vi "VFH Visualization.vi"() -> ()   [LabVIEW 2011]
uses:
  <vilib>/Platform/TimedLoop/XDataNode/timing_clust.ctl
  <vilib>/Platform/TimedLoop/XDataNode/nitl_modes.ctl
  <vilib>/Platform/TimedLoop/XDataNode/wakeup.ctl
  <vilib>/Platform/TimedLoop/XDataNode/XDataNode.xnode
  <vilib>/Platform/TimedLoop/XDataNode/XDNodeRunTimeDep.lvlib
  <vilib>/Analysis/NI_AALPro.lvlib
  <vilib>/Analysis/coordinate.llb/2D Cartesian Coordinate Rotation (Array).vi
  <vilib>/Analysis/NI_AAL_Angle.lvlib
  <vilib>/Analysis/coordinate.llb/Wrap Angle (scalar).vi
panel:
  in  "stop?":bool
  out "VY History":dbl(graph)
  out "Heading History":dbl(graph)
  out "LIDAR data":cluster{dbl[], dbl[]}[](graph)
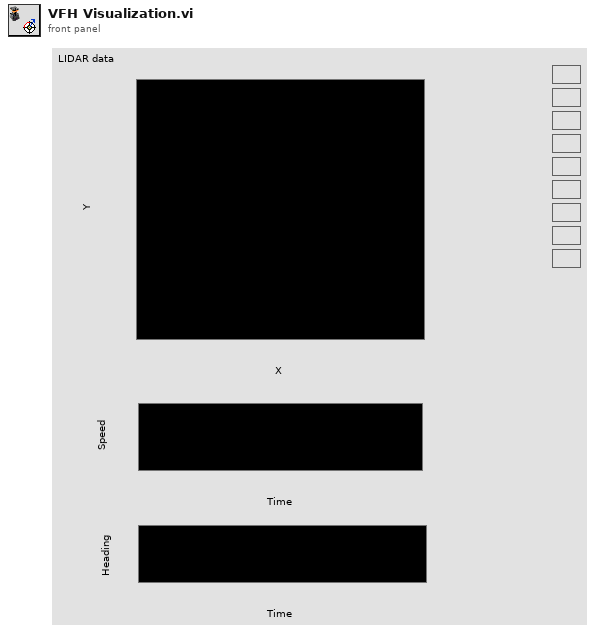
[diagram p1: front panel]
types:
  T1 = typedef "XDNodeRunTimeDep.lvlib/timing_clust.ctl" = cluster{"Expected End [f-1]":u64, "Actual End [f-1]":u64, "Finished Late? [f-1]":bool, "Expected End [i-1]":u64, "Actual End [i-1]":u64, "Finished Late? [i-1]":bool, "Expected Start [i]":u64, "Actual Start [i]":u64, "Expected Start [f]":u64, "Actual Start [f]":u64, "Source Name":string, "Structure Name":string, "Period":i64, "Deadline":i64, "Offset":i64, "Start":i64, "Priority":i32, "Timeout":i32, "Mode":T2, "Wakeup Reason":T3, "Error":errorcluster, "Source Type":string, "Secondary Source Type":string, "Global End Time":u64, "Global Start Time":u64, "Frame Duration":u64, "Iteration Duration":u64, "Assigned CPU":i32, "I/O Scan Engine Mode":u32}
  T2 = typedef "XDNodeRunTimeDep.lvlib/nitl_modes.ctl" = enum32{"No Change", "Process missed periods, maintain original phase", "Discard missed periods, maintain original phase", "Process missed periods, ignore original phase", "Discard missed periods, ignore original phase"}
  T3 = typedef "XDNodeRunTimeDep.lvlib/wakeup.ctl" = enum32{"Normal", "Aborted", "Asynchronous wakeup", "Timing source error", "Timed loop error", "Timeout"}
  T4 = cluster{"Latitude":dbl, "Longitude":dbl, "Altitude":dbl, "Velocity, Correction & SET":cluster{"Velocity North":dbl, "Velocity East":dbl, "Velocity Up":dbl, "Ellipsoidal Height":dbl, "GDOP":sgl, "PDOP":sgl, "HDOP":sgl, "VDOP":sgl, "TDOP":sgl, "Horizontal Figure of Merit":u8, "Time Figure of Merit":u8, "Max dGPS Age":sgl, "Extended Navigation Mode":u8, "Antenna Height Adjustment ":dbl, "SET North":i32, "SET East":i32, "SET Up":i32}, "Time":cluster{"GPS Week":u16, "GPS Time of Week":sgl}, "Satellites Used":i32[]}
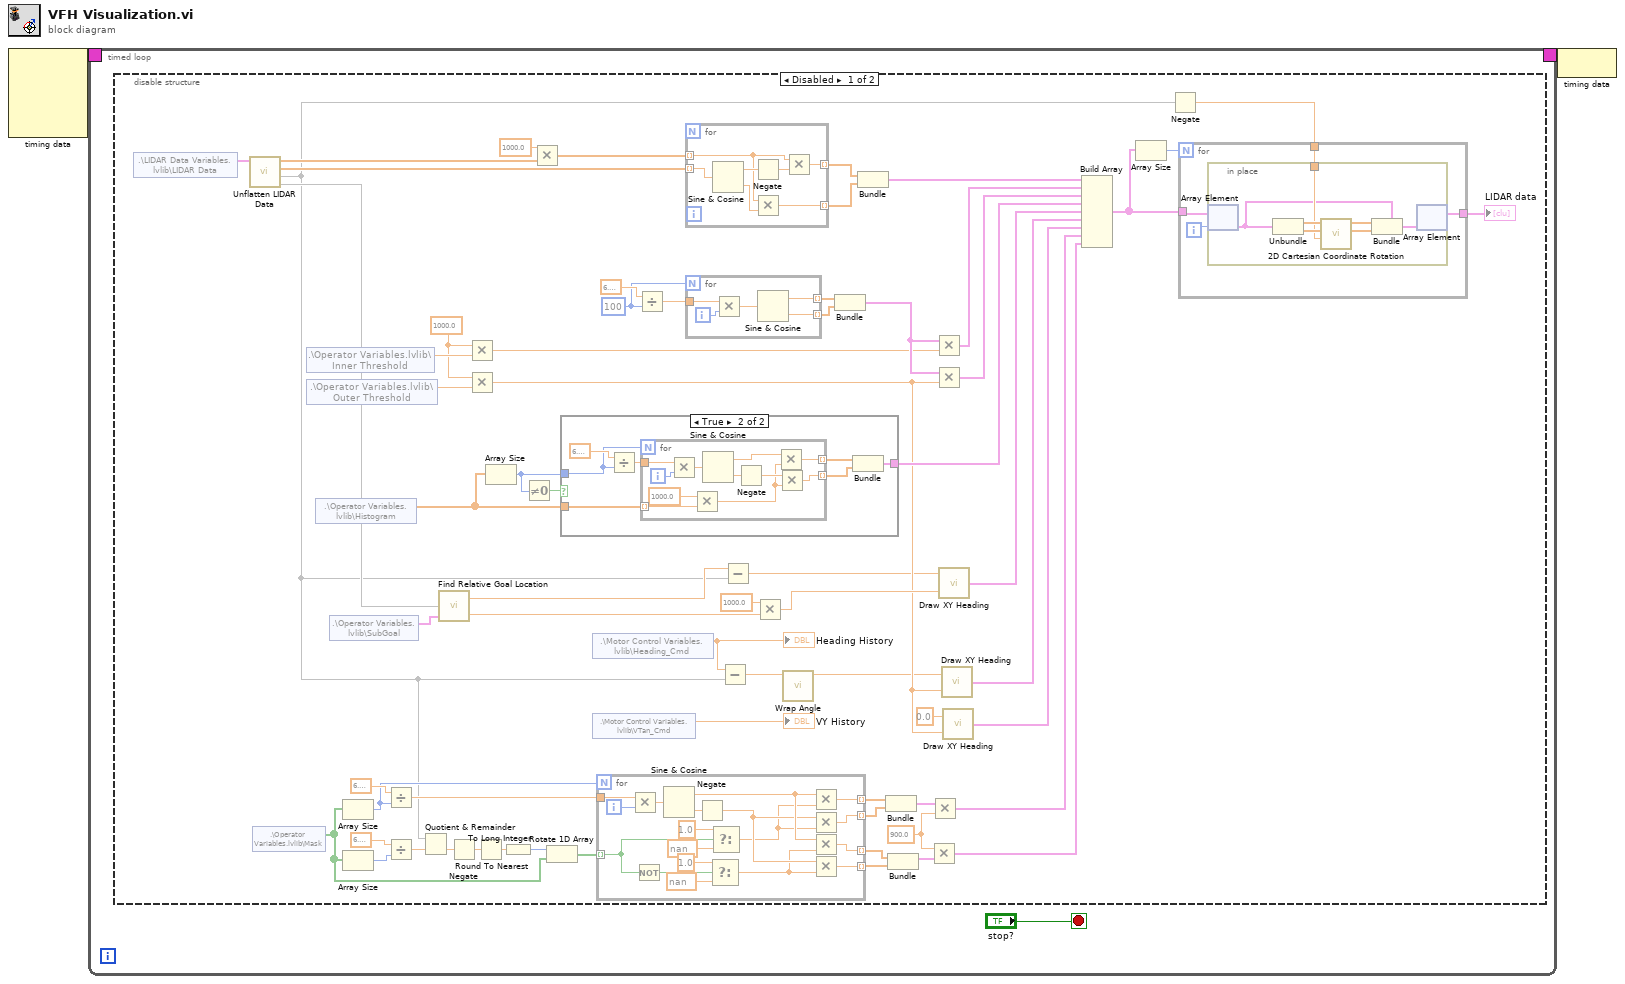
[diagram p0: block diagram]
diagram:
  n1 = node-c288() -> (w2:T1)  [unwired: 4 out]
  n2 = timed-loop {
    timing: w2 -> [_]
    timing-out: [_] -> w1
    stop <- "stop?" stop-if-true
    n3 = disable-structure shown="Disabled" {
      frame Disabled {
        w20 = 1000.0 ("x")
        w6 = 900.0 ("y")
        w67 = 100 ("y")
        n4 = shared-variable ".\\LIDAR Data Variables.lvlib\\LIDAR Data"() -> (w18:cluster{"Magnitude":dbl[], "Direction":dbl[]})  [unwired: 1 in, 1 out]
        n5 = call "Unflatten LIDAR Data.vi"("LIDAR Data"=w18) -> (0:w15, 1:w11, "Bearing (rad)"=w16:dbl[], "Range (m)"=w17:dbl[])  [unwired: 7 in]
        n6 = shared-variable ".\\Operator Variables.lvlib\\Mask"() -> (w36:bool[])  [unwired: 1 in, 1 out]
        n7 = shared-variable ".\\Operator Variables.lvlib\\Inner Threshold"() -> (w25:dbl)  [unwired: 1 in, 1 out]
        n8 = shared-variable ".\\Operator Variables.lvlib\\Outer Threshold"() -> (w24:dbl)  [unwired: 1 in, 1 out]
        n9 = shared-variable ".\\Operator Variables.lvlib\\Histogram"() -> (w41:dbl[])  [unwired: 1 in, 1 out]
        n10 = shared-variable ".\\Operator Variables.lvlib\\SubGoal"() -> (w40:T4)  [unwired: 1 in, 1 out]
        n11 = Array Size(array=w36) -> (size(s)=w59:i32)
        n12 = Array Size(array=w36) -> (size(s)=w51:i32)
        n13 = Divide(x=6.283185307179586, y=w59) -> (x/y=w60:dbl)
        n14 = Divide(x=6.283185307179586, y=w51) -> (x/y=w50:dbl)
        n15 = Quotient & Remainder(x=w11, y=w50) -> (floor(x/y)=w49:dbl)  [unwired: 1 out]
        n16 = call "Find Relative Goal Location.vi"("Goal Position 1"=w40, "Current Position 1"=w15) -> ("Target Distance"=w37:dbl, "Target Heading"=w12:dbl)  [unwired: 1 in]
        n17 = Negate(x=w49) -> (-x=w48:dbl)
        n18 = Multiply(x=w20, y=w25) -> (x*y=w22:dbl)
        n19 = Multiply(x=w20, y=w24) -> (x*y=w21:dbl)
        n20 = Round To Nearest(number=w48) -> (nearest integer value=w47:dbl)
        n21 = Array Size(array=w41) -> (size(s)=w35:i32)
        n22 = To Long Integer(number=w47) -> (32bit integer=w46:i32)
        n23 = Not Equal To 0?(x=w35) -> (x != 0?=w34:bool)
        n24 = Multiply(x=1000.0, y=w17) -> (x*y=w14:dbl[])
        n25 = Rotate 1D Array(1:w36, 2:w46) -> (0:w45:bool[])
        n26 = case shown="True" w34 {
          tunnel: [_ w76] -> w33
          tunnel: w41 -> [_ w71]
          tunnel: w35 -> [_ w70]
          frame False {
          }
          frame True {
            n27 = Divide(x=6.283185307179586, y=w70) -> (x/y=w73:dbl)
            n28 = for {
              N: w70 -> [_]
              tunnel: w73 -> [w86]
              tunnel: [w81] -> w74 mode=indexing
              tunnel: [w80] -> w75 mode=indexing
              tunnel: w71 -> [w79] mode=indexing
              i -> [w87]
              n29 = Multiply(x=w86, y=w87) -> (x*y=w85:dbl)
              n30 = Multiply(x=1000.0, y=w79) -> (x*y=w78:dbl)
              n31 = Sine & Cosine(0:w85) -> (1:w84:dbl, 2:w83:dbl)
              n32 = Negate(x=w83) -> (-x=w82:dbl)
              n33 = Multiply(x=w84, y=w78) -> (x*y=w81:dbl)
              n34 = Multiply(x=w82, y=w78) -> (x*y=w80:dbl)
            }
            n35 = Bundle(w74, w75) -> (w76:cluster{dbl[], dbl[]})  [unwired: 1 out]
          }
        }
        n36 = shared-variable ".\\Motor Control Variables.lvlib\\Heading_Cmd"() -> (w27:dbl)  [unwired: 1 in, 1 out]
        "Heading History" <- w27
        n37 = shared-variable ".\\Motor Control Variables.lvlib\\VTan_Cmd"() -> (→"VY History":dbl)  [unwired: 1 in, 1 out]
        n38 = for {
          N: w59 -> [_]
          tunnel: w60 -> [w111]
          tunnel: [w102] -> w57 mode=indexing
          tunnel: [w101] -> w56 mode=indexing
          tunnel: w45 -> [w104] mode=indexing
          tunnel: [w99] -> w55 mode=indexing
          tunnel: [w100] -> w54 mode=indexing
          i -> [w112]
          n39 = Multiply(x=w111, y=w112) -> (x*y=w110:dbl)
          n40 = Not(x=w104) -> (.not. x?=w103:bool)
          n41 = Sine & Cosine(0:w110) -> (1:w98:dbl, 2:w109:dbl)
          n42 = Negate(x=w109) -> (-x=w97:dbl)
          n43 = Select(t=1.0, s=w103, f=nan) -> (s? t:f=w95:dbl)
          n44 = Select(t=1.0, s=w104, f=nan) -> (s? t:f=w96:dbl)
          n45 = Multiply(x=w98, y=w96) -> (x*y=w102:dbl)
          n46 = Multiply(x=w97, y=w96) -> (x*y=w101:dbl)
          n47 = Multiply(x=w98, y=w95) -> (x*y=w99:dbl)
          n48 = Multiply(x=w97, y=w95) -> (x*y=w100:dbl)
        }
        n49 = Divide(x=6.283185307179586, y=w67) -> (x/y=w66:dbl)
        n50 = for {
          tunnel: w14 -> [w88] mode=indexing
          tunnel: w16 -> [w89] mode=indexing
          tunnel: [w92] -> w42 mode=indexing
          tunnel: [w91] -> w43 mode=indexing
          n51 = Sine & Cosine(0:w89) -> (1:w94:dbl, 2:w93:dbl)
          n52 = Negate(x=w94) -> (-x=w90:dbl)
          n53 = Multiply(x=w88, y=w93) -> (x*y=w91:dbl)
          n54 = Multiply(x=w88, y=w90) -> (x*y=w92:dbl)
        }
        n55 = for {
          N: w67 -> [_]
          tunnel: w66 -> [w127]
          tunnel: [w125] -> w65 mode=indexing
          tunnel: [w124] -> w64 mode=indexing
          i -> [w128]
          n56 = Multiply(x=w127, y=w128) -> (x*y=w126:dbl)
          n57 = Sine & Cosine(0:w126) -> (1:w125:dbl, 2:w124:dbl)
        }
        n58 = Subtract(x=w27, y=w11) -> (x-y=w5:dbl)
        n59 = Subtract(x=w12, y=w11) -> (x-y=w10:dbl)
        n60 = Multiply(x=1000.0 ("y"), y=w37) -> (x*y=w38:dbl)
        n61 = call-poly <vilib>:"Wrap Angle.vi"("angle in"=w5) -> ("angle out"=w4:dbl)  [unwired: 9 in, 1 out]
        n62 = Bundle(w65, w64) -> (w23:cluster{dbl[], dbl[]})  [unwired: 1 out]
        n63 = Bundle(w42, w43) -> (w69:cluster{dbl[], dbl[]})  [unwired: 1 out]
        n64 = Bundle(w57, w56) -> (w58:cluster{dbl[], dbl[]})  [unwired: 1 out]
        n65 = Bundle(w55, w54) -> (w53:cluster{dbl[], dbl[]})  [unwired: 1 out]
        n66 = Multiply(x=w6, y=w53) -> (x*y=w28:cluster{dbl[], dbl[]})
        n67 = Multiply(x=w58, y=w6) -> (x*y=w29:cluster{dbl[], dbl[]})
        n68 = Multiply(x=w23, y=w22) -> (x*y=w26:cluster{dbl[], dbl[]})
        n69 = Multiply(x=w23, y=w21) -> (x*y=w63:cluster{dbl[], dbl[]})
        n70 = call "Draw XY Heading.vi"("Length"=w38, "Direction"=w10) -> ("Heading Graph"=w32:cluster{dbl[], dbl[]})
        n71 = call "Draw XY Heading.vi"("Length"=w21, "Direction"=w4) -> ("Heading Graph"=w31:cluster{dbl[], dbl[]})
        n72 = call "Draw XY Heading.vi"("Length"=w21, "Direction"=0.0) -> ("Heading Graph"=w30:cluster{dbl[], dbl[]})
        n73 = Build Array(w69, w26, w63, w33, w32, w31, w30, w29, w28) -> (w8:cluster{dbl[], dbl[]}[])
        n74 = Array Size(array=w8) -> (size(s)=w7:i32)
        n75 = Negate(x=w11) -> (-x=w62:dbl)
        n76 = for {
          N: w7 -> [_]
          tunnel: w8 -> [w115]
          tunnel: w62 -> [w116]
          tunnel: [w114] -> w9
          i -> [w113]
          n77 = in-place {
            in-place-border: w116 -> [w119]
            n78 = in-place-array #1(w115, w113) -> (w118:cluster{dbl[], dbl[]})
            n79 = Unbundle(w118) -> (w123:dbl[], w122:dbl[])
            n80 = call-poly <vilib>:"2D Cartesian Coordinate Rotation.vi"("theta"=w119, "Y"=w122, "X"=w123) -> ("Y Out"=w120:dbl[], "X Out"=w121:dbl[])  [unwired: 6 in, 1 out]
            n81 = Bundle(cluster=w118, w121, w120) -> (w117:cluster{dbl[], dbl[]})
            n82 = in-place-array #1(w117) -> (w114:cluster{dbl[], dbl[]}[])  [unwired: 1 out]
          }
        }
        "LIDAR data" <- w9
      }
      frame Enabled {
      }
    }
  }
  n83 = node-c288(w1) -> ()
